vi "Finish.vi"   [LabVIEW 2019]
doc: "This VI is called just before exiting. It is expected to close I/O refnum, save collected data, etc."
uses:
  <vilib>/Rock Robotics/WPI/Utilities/WPI_GetSetVariantRefNum.vi
types:
  T1 = typedef "WPI_MotorControlDeviceRef.ctl" = cluster{"DeviceStatus":errorcluster, "Type":T2, "PWM":cluster{"PWM Channel":T3, "DeadBand":T4}, "CAN":cluster{"Device Number":u8, "SetOutput VI Ref":variant, "GetOutput VI Ref":variant, "Enable VI Ref":variant, "Disable VI Ref":variant, "Data":variant}, "Invert":bool, "DIO PWM":cluster{"PWM \"Enable\" Channel":T3, "DIOChannel":T5, "PWM Rate":dbl}}
  T2 = typedef "WPI_MotorControlType.ctl" = enum16{"PWM", "CAN", "DIO PWM"}
  T3 = typedef "FPGA_DIOPWMChannel.ctl" = enum8{"PWM 0", "PWM 1", "PWM 2", "PWM 3", "PWM 4", "PWM 5", "PWM 6", "PWM 7", "PWM 8", "PWM 9", "PWM MXP 0", "PWM MXP 1", "PWM MXP 2", "PWM MXP 3", "PWM MXP 4", "PWM MXP 5", "PWM MXP 6", "PWM MXP 7", "PWM MXP 8", "PWM MXP 9", "Invalid"}
  T4 = typedef "WPI_PWMDeadband.ctl" = cluster{"Name":string, "maxPositivePwm":i32, "minPositivePwm":i32, "centerPwm":i32, "maxNegativePwm":i32, "minNegativePwm":i32, "angularRange":u16}
  T5 = typedef "FPGA_DIOChannel.ctl" = enum8{"DIO 0", "DIO 1", "DIO 2", "DIO 3", "DIO 4", "DIO 5", "DIO 6", "DIO 7", "DIO 8", "DIO 9", "DIO MXP 0", "DIO MXP 1", "DIO MXP 2", "DIO MXP 3", "DIO MXP 4", "DIO MXP 5", "DIO MXP 6", "DIO MXP 7", "DIO MXP 8", "DIO MXP 9", "DIO MXP 10", "DIO MXP 11", "DIO MXP 12", "DIO MXP 13", "DIO MXP 14", "DIO MXP 15", "SPI Port CS1", "SPI Port CS2", "SPI Port CS3", "SPI Port MISO", "SPI Port MOSI", "Invalid"}
  T6 = typedef "WPI_SwitchDevRef.ctl" = cluster{"DevStatus":errorcluster, "DIO Channel":T5, "CntIndex":T7, "Normally Closed":bool}
  T7 = typedef "FPGA_CounterCtrSystemIndex.ctl" = enum8{"Ctr 0", "Ctr 1", "Ctr 2", "Ctr 3", "Ctr 4", "Ctr 5", "Ctr 6", "Ctr 7", "Invalid"}
  T8 = typedef "WPI_JoystickDevRef.ctl" = cluster{"Device":T9}
  T9 = typedef "WPI_JoystickDeviceEnum.ctl" = enum16{"USB 0", "USB 1", "USB 2", "USB 3", "USB 4", "USB 5"}
  T10 = typedef "WPI_RobotDriveDevRef.ctl" = cluster{"DevStatus":errorcluster, "Motors[]":T1[], "Square Inputs":bool, "Max Output":dbl}
  T11 = typedef "WPI_GyroDevRef.ctl" = cluster{"DevStatus":errorcluster, "Analog Channel":T12, "Gain (VoltsPerDegree/Second)":dbl, "Gyro Type":enum16{"Analog", "XRS450"}, "Handle":i32, "SPI Bus":T13, "Device Found":bool, "Sample Rate":dbl, "Calibrate On Open":bool, "Offset":dbl}
  T12 = typedef "FPGA_AIChannel.ctl" = enum8{"AI 0", "AI 1", "AI 2", "AI 3", "AI MXP 0", "AI MXP 1", "AI MXP 2", "AI MXP 3", "Invalid"}
  T13 = typedef "spi_bus.ctl" = enum16{"SPI On-Board, CS0", "SPI On-Board, CS1", "SPI On-Board, CS2", "SPI On-Board, CS3", "SPI MXP", "Invalid"}
  T14 = typedef "WPI_AnalogChannelDevRef.ctl" = cluster{"DevStatus":errorcluster, "Analog Channel":T12}
  T15 = typedef "WPI_DigitalOutputDevRef.ctl" = cluster{"DIO Channel":T5, "DevStatus":errorcluster}
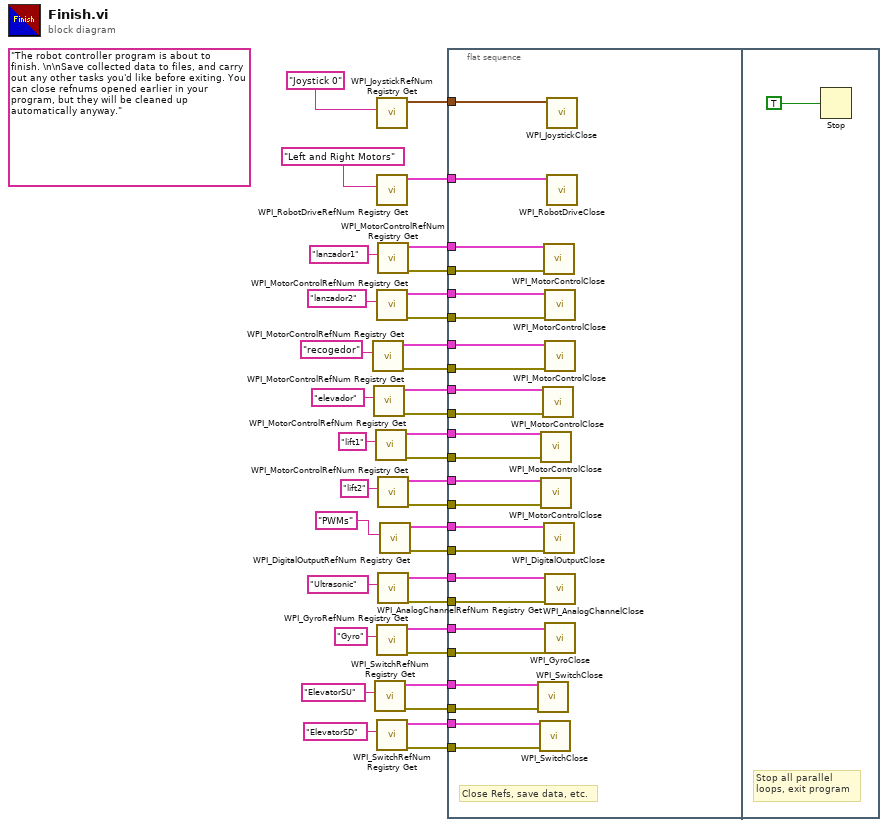
[diagram p0: block diagram]
diagram:
  (unwired) "The robot controller program is about to finish. \n\nSave collected data to files, and carry out any other tasks you'd like before exiting. You can close refnums opened earlier in your program, but they will be cleaned up automatically anyway."
  n1 = call <vilib>:"WPI_MotorControlRefNum Registry Get.vi"("refnum name"="recogedor") -> ("error out"=w25:errorcluster, "MotorControlDevRef"=w26:T1)  [unwired: 9 in]
  n2 = call <vilib>:"WPI_MotorControlRefNum Registry Get.vi"("refnum name"="elevador") -> ("error out"=w17:errorcluster, "MotorControlDevRef"=w18:T1)  [unwired: 9 in]
  n3 = call <vilib>:"WPI_SwitchRefNum Registry Get.vi"("refnum name"="ElevatorSU") -> ("error out"=w3:errorcluster, "SwitchDevRef"=w4:T6)  [unwired: 9 in]
  n4 = call <vilib>:"WPI_MotorControlRefNum Registry Get.vi"("refnum name"="lift1") -> ("error out"=w11:errorcluster, "MotorControlDevRef"=w12:T1)  [unwired: 9 in]
  n5 = call <vilib>:"WPI_JoystickRefNum Registry Get.vi"("refnum name"="Joystick 0") -> ("JoystickDevRef"=w34:T8)  [unwired: 1 in, 9 out]
  n6 = call <vilib>:"WPI_RobotDriveRefNum Registry Get.vi"("refnum name"="Left and Right Motors") -> ("RobotDriveDevRef"=w35:T10)  [unwired: 1 in, 9 out]
  n7 = call <vilib>:"WPI_MotorControlRefNum Registry Get.vi"("refnum name"="lanzador2") -> ("error out"=w28:errorcluster, "MotorControlDevRef"=w29:T1)  [unwired: 9 in]
  n8 = call <vilib>:"WPI_GyroRefNum Registry Get.vi"("refnum name"="Gyro") -> ("error out"=w20:errorcluster, "GyroDevRef"=w21:T11)  [unwired: 9 in]
  n9 = call <vilib>:"WPI_SwitchRefNum Registry Get.vi"("refnum name"="ElevatorSD") -> ("error out"=w1:errorcluster, "SwitchDevRef"=w2:T6)  [unwired: 9 in]
  n10 = call <vilib>:"WPI_MotorControlRefNum Registry Get.vi"("refnum name"="lanzador1") -> ("error out"=w32:errorcluster, "MotorControlDevRef"=w33:T1)  [unwired: 9 in]
  n11 = call <vilib>:"WPI_MotorControlRefNum Registry Get.vi"("refnum name"="lift2") -> ("error out"=w14:errorcluster, "MotorControlDevRef"=w15:T1)  [unwired: 9 in]
  n12 = call <vilib>:"WPI_AnalogChannelRefNum Registry Get.vi"("refnum name"="Ultrasonic") -> ("error out"=w23:errorcluster, "AIDeviceRef"=w24:T14)  [unwired: 9 in]
  n13 = call <vilib>:"WPI_DigitalOutputRefNum Registry Get.vi"("refnum name"="PWMs") -> ("error out"=w7:errorcluster, "DigitalOutputDevRef"=w8:T15)  [unwired: 9 in]
  n14 = flat-sequence {
    tunnel: w35 -> [w61]
    tunnel: w34 -> [w60]
    tunnel: w33 -> [w59]
    tunnel: w32 -> [w58]
    tunnel: w29 -> [w57]
    tunnel: w28 -> [w56]
    tunnel: w26 -> [w55]
    tunnel: w25 -> [w54]
    tunnel: w24 -> [w53]
    tunnel: w23 -> [w52]
    tunnel: w21 -> [w51]
    tunnel: w20 -> [w50]
    tunnel: w18 -> [w49]
    tunnel: w17 -> [w48]
    tunnel: w15 -> [w47]
    tunnel: w14 -> [w46]
    tunnel: w12 -> [w45]
    tunnel: w11 -> [w44]
    tunnel: w8 -> [w43]
    tunnel: w7 -> [w42]
    tunnel: w4 -> [w41]
    tunnel: w3 -> [w40]
    tunnel: w2 -> [w39]
    tunnel: w1 -> [w38]
    frame #0 {
      # "Close Refs, save data, etc."
      n15 = call <vilib>:"WPI_SwitchClose.vi"("error in (no error)"=w40, "SwitchDevRef"=w41) -> ()  [unwired: 9 in, 1 out]
      n16 = call <vilib>:"WPI_SwitchClose.vi"("error in (no error)"=w38, "SwitchDevRef"=w39) -> ()  [unwired: 9 in, 1 out]
      n17 = call <vilib>:"WPI_MotorControlClose.vi"("error in"=w44, "MotorControlDevRef"=w45) -> ()  [unwired: 9 in, 1 out]
      n18 = call <vilib>:"WPI_MotorControlClose.vi"("error in"=w46, "MotorControlDevRef"=w47) -> ()  [unwired: 9 in, 1 out]
      n19 = call <vilib>:"WPI_MotorControlClose.vi"("error in"=w48, "MotorControlDevRef"=w49) -> ()  [unwired: 9 in, 1 out]
      n20 = call <vilib>:"WPI_MotorControlClose.vi"("error in"=w58, "MotorControlDevRef"=w59) -> ()  [unwired: 9 in, 1 out]
      n21 = call <vilib>:"WPI_DigitalOutputClose.vi"("error in (no error)"=w42, "DigitalOutputDevRef"=w43) -> ()  [unwired: 9 in, 1 out]
      n22 = call <vilib>:"WPI_MotorControlClose.vi"("error in"=w56, "MotorControlDevRef"=w57) -> ()  [unwired: 9 in, 1 out]
      n23 = call <vilib>:"WPI_MotorControlClose.vi"("error in"=w54, "MotorControlDevRef"=w55) -> ()  [unwired: 9 in, 1 out]
      n24 = call <vilib>:"WPI_AnalogChannelClose.vi"("error in (no error)"=w52, "AIDeviceRef"=w53) -> ()  [unwired: 9 in, 1 out]
      n25 = call <vilib>:"WPI_GyroClose.vi"("error in"=w50, "GyroDevRef"=w51) -> ()  [unwired: 9 in, 1 out]
      n26 = call <vilib>:"WPI_JoystickClose.vi"("JoystickDevRef"=w60) -> ()  [unwired: 11 out]
      n27 = call <vilib>:"WPI_RobotDriveClose.vi"("RobotDriveDevRef"=w61) -> ()  [unwired: 1 in, 10 out]
    }
    frame #1 {
      # "Stop all parallel\nloops, exit program"
      n28 = Stop(stop? (T)=TRUE ("Quit")) -> ()
    }
  }
